vi "discover_devices.vi"(8 "error in (no error)":errorcluster, 11 "device filter":string(combo)="all") -> (0 "error out":errorcluster, 1 "nbr of found devices":i32, 2 "Device-Infos":T1(array[cluster]), 3 "IP-Addresses":string[](array[string]))   [LabVIEW 2016, in "sen_api.lvlib"]
uses:
  <vilib>/nisyscfg/Close (System).vi
  <vilib>/Utility/tcp.llb/UDP Multicast Read-Write Open.vi
  sen_api.lvlib
  <vilib>/httpClient/LabVIEWHTTPClient.lvlib
  <vilib>/nisyscfg/nisyscfg.lvlib
  <resource>/objmgr/nisysapi.rc
panel:
  in  "dev-Info-fields":string[](array[string])=["ipAddress", "modelName", "serialNumber", "friendlyName", "macAddress", "lockedStatus"]
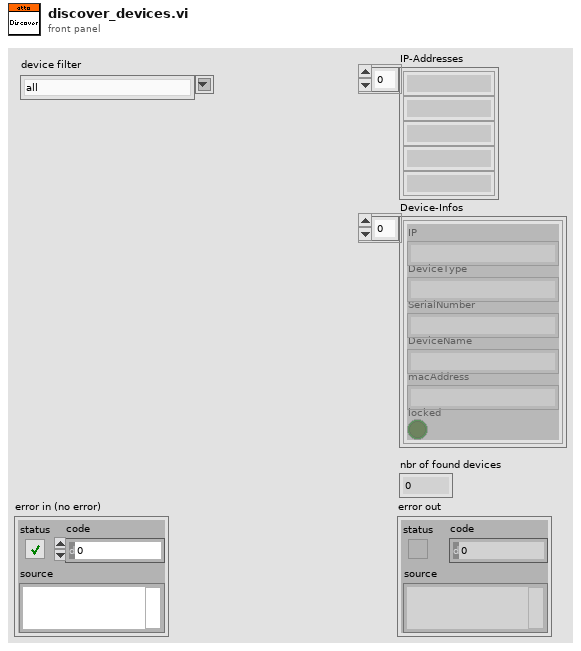
[diagram p1: front panel]
types:
  T1 = cluster{"IP":string, "DeviceType":string, "SerialNumber":string, "DeviceName":string, "macAddress":string, "locked":bool}[]
  T2 = cluster{"IP":string, "DeviceType":string, "SerialNumber":string, "DeviceName":string, "macAddress":string, "locked":bool}
  T3 = typedef "LabVIEWHTTPClient.lvlib/ClientHandle.ctl" = refnum<k1>
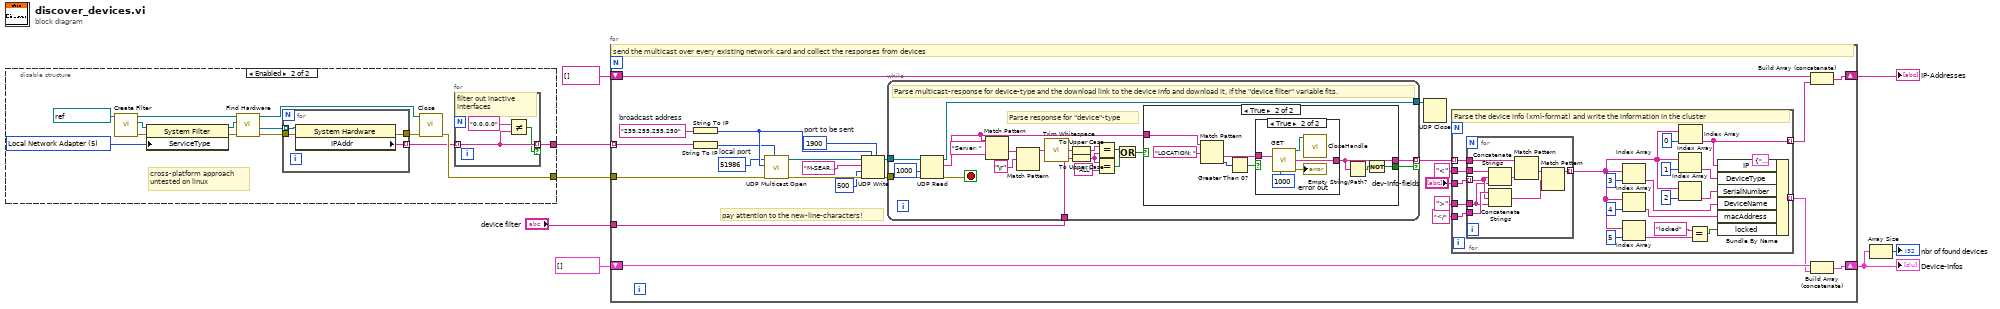
[diagram p0: block diagram]
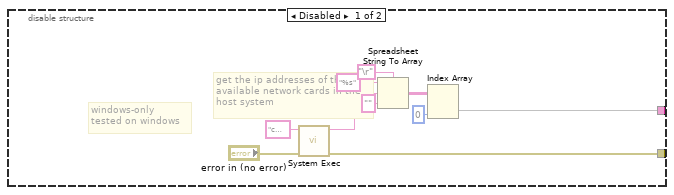
[diagram p2: hidden frame]
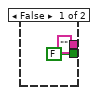
[diagram p3: hidden frame]
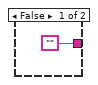
[diagram p4: hidden frame]
diagram:
  n1 = disable-structure shown="Enabled" {
    disable-tunnel: [w11 w19] -> w8
    disable-tunnel: [w10 w21] -> w2
    frame Disabled {
      # "windows-only\ntested on windows"
      # "get the ip addresses of the\navailable network cards in the\nhost system"
      n2 = call <vilib>:"System Exec.vi"("error in (no error)"="error in (no error)", "command line"="cmd /c for /F \"tokens=14 delims= \" %i in ('ipconfig ^| findstr /R /C:\"IPv4 Address\"') do @echo %i") -> ("error out"=w10:errorcluster, "standard output"=w17:string)  [unwired: 6 in, 2 out]
      n3 = Spreadsheet String To Array(delimiter (Tab)="\r", format string="%s", spreadsheet string=w17, array type (2D Dbl)="") -> (array=w13:string[][])
      n4 = Index Array(array=w13, index (col)=0 ("disabled index (col)")) -> (element=w11:string[])  [unwired: 1 in]
    }
    frame Enabled {
      w27 = u32 5 items=["NI Network Resource", "NI Real-Time", "NI System Configuration", "NI Web Interface", "Local System", "Local Network Adapter", "Local Time Keeper", "Local Time Reference", "LXI Instrument", "Local FPGA"] ("Service Type")
      # "cross-platform approach\nuntested on linux"
      n5 = call <vilib>:"Create Filter.vi"("Session in"=refnum<k21> "localhost" ("System Configuration")) -> ("error out"=w23:errorcluster, "Filter out"=w24:refnum<k20>, "Session out"=w26:refnum<k21>)  [unwired: 8 in]
      n6 = property class="System Filter"(reference=w24, error in=w23, "ServiceType"=w27) -> (reference out=w28:refnum<k20>, error out=w29:errorcluster)
      n7 = call <vilib>:"Find Hardware.vi"("error in (no error)"=w29, "Filter in"=w28, "Session in"=w26) -> ("error out"=w30:errorcluster, "Resources out"=w22:refnum<k20>[], "Session out"=w32:refnum<k21>)  [unwired: 5 in, 1 out]
      n8 = for {
        tunnel: w22 -> [w38] mode=indexing
        tunnel: [w39] -> w20 mode=indexing
        tunnel: w30 -> [w37]
        tunnel: [w36] -> w31
        n9 = property class="System Hardware"(reference=w38, error in=w37) -> (error out=w36:errorcluster, "IPAddr"=w39:string)  [unwired: 1 out]
      }
      n10 = call-poly <vilib>:"Close.vi"("error in (no error)"=w31, "Session in"=w32) -> ("error out"=w21:errorcluster)  [unwired: 9 in]
      n11 = for {
        tunnel: w20 -> [w35] mode=indexing
        tunnel: [w35] -> w19 mode=indexing if=w33
        # "filter out inactive\ninterfaces"
        n12 = Not Equal?(x="0.0.0.0", y=w35) -> (x != y?=w33:bool)
      }
    }
  }
  n13 = for {
    tunnel: w8 -> [w52] mode=indexing
    shift-right: [w49] -> w4
    shift-left: T1 [] -> [w51]
    shift-right: [w48] -> w5
    shift-left: string[] [] -> [w46]
    tunnel: w2 -> [w45]
    tunnel: "device filter" -> [w41]
    w61 = u16 1900  # port to be sent
    w55 = u16 51986  # local port
    w65 = "239.255.255.250"  # broadcast address
    # "pay attention to the new-line-characters!"
    # "send the multicast over every existing network card and collect the responses from devices"
    n14 = String To IP(1:w65) -> (0:w62:u32)
    n15 = String To IP(1:w52) -> (0:w54:u32)
    n16 = call-poly <vilib>:"UDP Multicast Open.vi"("net address"=w54, "error in (no error)"=w45, "multicast addr"=w62, "port"=w55) -> ("error out"=w44:errorcluster, "connection ID"=w64:refnum<k16>)  [unwired: 5 in, 1 out]
    n17 = UDP Write(address=w62, port or service name=w61, connection ID=w64, data in="M-SEARCH * HTTP/1.1\r\nHOST: 239.255.255.250:1900\r\nST: ssdp:all\r\nMAN: \"ssdp:discover\"\r\nMX: 3\r\n\r\n", 8:w44, 9:500 ("timeout ms (25000)")) -> (error out=w42:errorcluster, 3:w60:refnum<k16>)
    n18 = while {
      tunnel: [w85] -> w63
      tunnel: w60 -> [w84]
      tunnel: [w81] -> w40 mode=indexing if=w80
      tunnel: w42 -> [w79]
      tunnel: w41 -> [w74]
      stop <- w82 stop-if-true
      # "Parse response for \"device\"-type"
      # "Parse multicast-response for device-type and the download link to the device info and download it, if the \"device filter\" variable fits."
      n19 = UDP Read(connection ID=w84, timeout ms (25000)=1000 ("max size (548)"), 8:w79) -> (data out=w75:string, error out=w82:errorcluster, 3:w85:refnum<k16>)  [unwired: 1 in, 2 out]
      n20 = Match Pattern(string=w75, regular expression="Server: ") -> (after substring=w77:string)  [unwired: 1 in, 3 out]
      n21 = Match Pattern(string=w77, regular expression="\r") -> (before substring=w73:string)  [unwired: 1 in, 3 out]
      n22 = call <vilib>:"Trim Whitespace.vi"("string"=w73) -> ("trimmed string"=w72:string)  [unwired: 1 in]
      n23 = To Upper Case(1:w72) -> (0:w70:string)
      n24 = To Upper Case(1:w74) -> (0:w68:string)
      n25 = Equal?(x=w70, y=w68) -> (x = y?=w69:bool)
      n26 = Equal?(x=w68, y="ALL" ("regular expression")) -> (x = y?=w66:bool)
      n27 = Or(x=w69, y=w66) -> (x .or. y?=w71:bool)
      n28 = case shown="True" w71 {
        tunnel: ["" ("body") w91] -> w81
        tunnel: [FALSE w89] -> w80
        tunnel: w75 -> [_ w88]
        frame False {
        }
        frame True {
          n29 = Match Pattern(string=w88, regular expression="LOCATION: ") -> (after substring=w92:string, offset past match=w94:i32)  [unwired: 1 in, 2 out]
          n30 = Greater Than 0?(x=w94) -> (x > 0?=w95:bool)
          n31 = case shown="True" w95 {
            tunnel: w92 -> [_ w100]
            tunnel: ["" w99] -> w91
            frame False {
            }
            frame True {
              n32 = call <vilib>:"GET.vi"("url"=w100, "timeout (10000)"=1000) -> ("client handle out"=w101:T3, "body"=w99:string, "error out"=→"error out":errorcluster)  [unwired: 10 in, 1 out]
              n33 = call <vilib>:"CloseHandle.vi"("client handle"=w101) -> ()  [unwired: 14 in, 1 out]
            }
          }
          n34 = Empty String/Path?(string/path=w91) -> (empty?=w90:bool)
          n35 = Not(x=w90) -> (.not. x?=w89:bool)
        }
      }
    }
    n36 = UDP Close(connection ID=w63) -> ()  [unwired: 1 in, 2 out]
    n37 = for {
      tunnel: w40 -> [w123] mode=indexing
      tunnel: "<" -> [w122]
      tunnel: ">" -> [w121]
      tunnel: "dev-Info-fields" -> [w120]
      tunnel: "</" -> [w102]
      tunnel: [w104] -> w50 mode=indexing
      tunnel: [w103] -> w47 mode=indexing
      # "Parse the device info (xml-format) and write the information in the cluster"
      n38 = for {
        tunnel: w123 -> [w132]
        tunnel: [w130] -> w118 mode=indexing
        tunnel: w122 -> [w129]
        tunnel: w121 -> [w125]
        tunnel: w120 -> [w126] mode=indexing
        tunnel: w102 -> [w127]
        n39 = Concatenate Strings(w129, w126, w125) -> (w128:string)
        n40 = Concatenate Strings(w127, w126, w125) -> (w124:string)
        n41 = Match Pattern(string=w132, regular expression=w128) -> (after substring=w131:string)  [unwired: 1 in, 3 out]
        n42 = Match Pattern(string=w131, regular expression=w124) -> (before substring=w130:string)  [unwired: 1 in, 3 out]
      }
      n43 = Index Array(array=w118, index=3) -> (element=w107:string)
      n44 = Index Array(array=w118, index=4) -> (element=w108:string)
      n45 = Index Array(array=w118, index=5) -> (element=w111:string)
      n46 = Index Array(array=w118, index=1) -> (element=w105:string)
      n47 = Index Array(array=w118, index=2) -> (element=w106:string)
      n48 = Index Array(array=w118, index=0) -> (element=w103:string)
      n49 = Equal?(x="locked", y=w111) -> (x = y?=w109:bool)
      n50 = Bundle By Name(cluster=T2 {"IP"="", "DeviceType"="", "SerialNumber"="", "DeviceName"="", "macAddress"="", "locked"=FALSE} ("DeviceInfo"), "IP"=w103, "DeviceType"=w105, "SerialNumber"=w106, "DeviceName"=w107, "macAddress"=w108, "locked"=w109) -> (w104:T2)
    }
    n51 = Build Array (concatenate)(w46, w47) -> (w48:string[])
    n52 = Build Array (concatenate)(w51, w50) -> (w49:T1)
  }
  "Device-Infos" <- w4
  "IP-Addresses" <- w5
  n53 = Array Size(array=w4) -> (size(s)=→"nbr of found devices":i32)
